vi "Set_speed_and_move_XY.vi"() -> ()   [LabVIEW 2013]
panel:
  out "Received String2 2":string="R\r\n"
  out "String Received 4":string="OK\r\n"
  out "Command String 4":string="A:2+P10000"
  out "OK move 2":bool=TRUE
  in  "Pulse Number 2":u32=10000 min=1 max=500000
  in  "Axis Number 2":u8=2
  out "OK speed 2":bool=TRUE
  out "String Received 3":string="OK\r\n"
  out "Command String 3":string="D:2S1000F10000R100"
  in  "Acceleration Time 2":u16=100 max=1000
  in  "High Speed 2":u32=10000 min=1 max=500000
  in  "Low Speed 2":u32=1000 min=1 max=500000
  out "Received String2":string="R\r\n"
  out "String Received 2":string="OK\r\n"
  out "Command String 2":string="A:1+P10000"
  out "OK move 1":bool=TRUE
  in  "Pulse Number 1":u32=10000 min=1 max=500000
  in  "Axis Number 1":u8=1
  out "OK speed 1":bool=TRUE
  in  "Port Number":i8=7 min=0
  out "String Received":string="OK\r\n"
  out "Command String":string="D:1S1000F10000R100"
  in  "Acceleration Time":u16=100 max=1000
  in  "High Speed":u32=10000 min=1 max=500000
  in  "Low Speed":u32=1000 min=1 max=500000
  # "For tensile test (30 mm sample length):\nSet local origin as X (axis 1) 27000, Y (axis 2) 5000"
  # "Set speed"
  # "Move to the absolute position"
  # "Abs. position X\nin um"
  # "X"
  # "Abs. position Y\nin um"
  # "Y"
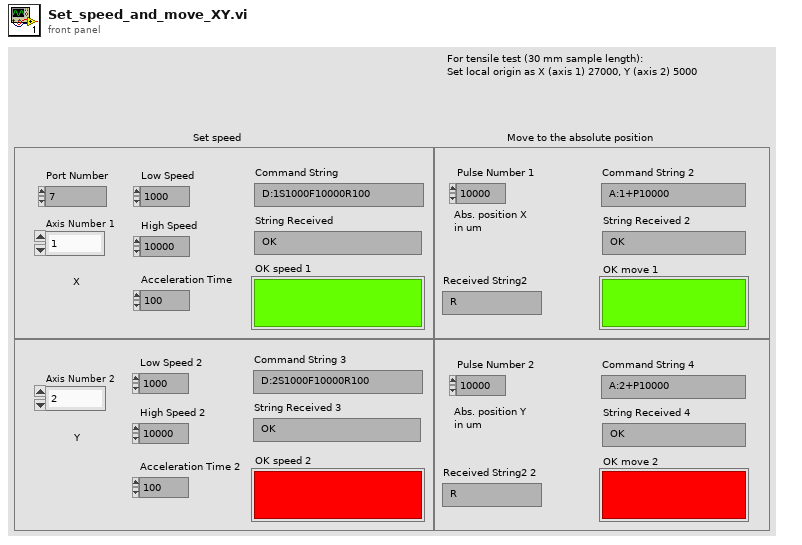
[diagram p1: front panel]
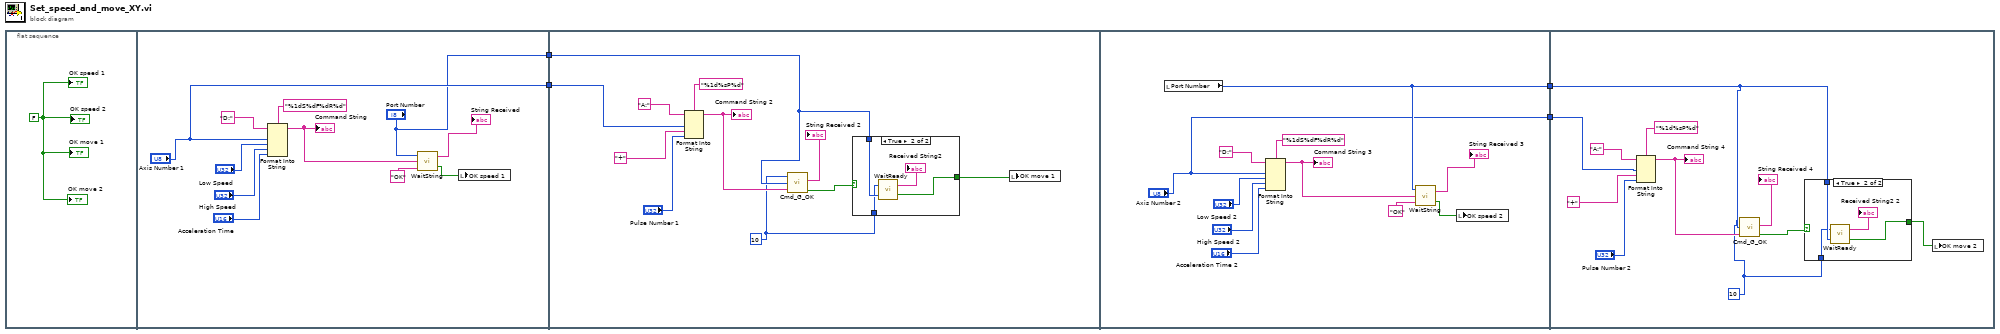
[diagram p0: block diagram]
diagram:
  n1 = flat-sequence {
    tunnel: ["Axis Number 1"] -> w4
    tunnel: ["Port Number"] -> w3
    tunnel: w4 -> [w20]
    tunnel: w3 -> [w19]
    tunnel: [w35] -> w2
    tunnel: ["Axis Number 2"] -> w1
    tunnel: w2 -> [w47]
    tunnel: w1 -> [w46]
    frame #0 {
      w5 = FALSE
      "OK speed 1" <- w5
      "OK speed 2" <- w5
      "OK move 1" <- w5
      "OK move 2" <- w5
    }
    frame #1 {
      n2 = Format Into String(format string="%1dS%dF%dR%d", initial string="D:", "Axis Number 1", "Low Speed", "High Speed", "Acceleration Time") -> (resulting string=w10:string)  [unwired: 1 in, 1 out]
      "Command String" <- w10
      n3 = call "WaitString.vi"("String to Receive"="OK", "String to Send"=w10, "PortNumber"="Port Number") -> ("OK Done"=w6:bool, "String Received"=→"String Received":string)
      n4 = local write "OK speed 1"(w6) -> ()
    }
    frame #2 {
      w17 = 10
      n5 = Format Into String(format string="%1d%sP%d", initial string="A:", w20, "+", "Pulse Number 1") -> (resulting string=w24:string)  [unwired: 1 in, 1 out]
      "Command String 2" <- w24
      n6 = call "Cmd_G_OK.vi"("Residence time"=w17, "PortNumber"=w19, "Command String"=w24) -> ("Received String2"=→"String Received 2":string, "OK Done"=w26:bool)  [unwired: 2 out]
      n7 = case shown="True" w26 {
        selector: w26 -> [w28 _]
        tunnel: w19 -> [_ w32]
        tunnel: [w28 w30] -> w18
        tunnel: w17 -> [_ w29]
        frame False {
        }
        frame True {
          n8 = call "WaitReady.vi"("PortNumber"=w32, "Residence time in ms"=w29) -> ("OK Done"=w30:bool, "String Received"=→"Received String2":string)
        }
      }
      n9 = local write "OK move 1"(w18) -> ()
    }
    frame #3 {
      n10 = local read "Port Number"() -> (w35:i8)
      n11 = Format Into String(format string="%1dS%dF%dR%d", initial string="D:", "Axis Number 2", "Low Speed 2", "High Speed 2", "Acceleration Time 2") -> (resulting string=w42:string)  [unwired: 1 in, 1 out]
      "Command String 3" <- w42
      n12 = call "WaitString.vi"("String to Receive"="OK", "String to Send"=w42, "PortNumber"=w35) -> ("OK Done"=w33:bool, "String Received"=→"String Received 3":string)
      n13 = local write "OK speed 2"(w33) -> ()
    }
    frame #4 {
      w44 = 10
      n14 = Format Into String(format string="%1d%sP%d", initial string="A:", w46, "+", "Pulse Number 2") -> (resulting string=w51:string)  [unwired: 1 in, 1 out]
      "Command String 4" <- w51
      n15 = call "Cmd_G_OK.vi"("Residence time"=w44, "PortNumber"=w47, "Command String"=w51) -> ("Received String2"=→"String Received 4":string, "OK Done"=w49:bool)  [unwired: 2 out]
      n16 = case shown="True" w49 {
        selector: w49 -> [w55 _]
        tunnel: [w55 w58] -> w45
        tunnel: w47 -> [_ w57]
        tunnel: w44 -> [_ w56]
        frame False {
        }
        frame True {
          n17 = call "WaitReady.vi"("PortNumber"=w57, "Residence time in ms"=w56) -> ("OK Done"=w58:bool, "String Received"=→"Received String2 2":string)
        }
      }
      n18 = local write "OK move 2"(w45) -> ()
    }
  }
